vi "findChannelByAddress.vi"(8 "error in (no error)":errorcluster, 10 "channel_address":string, 11 "DeviceArray in":refnum<class "DeviceArray.lvclass">) -> (0 "error out":errorcluster, 1 "Channel.lvclass":refnum<class "Channel.lvclass">, 2 "device.lvclass":refnum<class "device.lvclass">, 3 "DeviceArray out":refnum<class "DeviceArray.lvclass">, 4 "found?":bool)   [LabVIEW 2011, in "Tools.lvlib" / "DatabaseHelpers.lvlib" / "DeviceArray.lvclass"]
uses:
  DeviceArray.lvclass
  Channel/Channel.lvclass
  device/device.lvclass
  DeviceArray.lvclass/DeviceArray.ctl
  ChannelArray/ChannelArray.lvclass
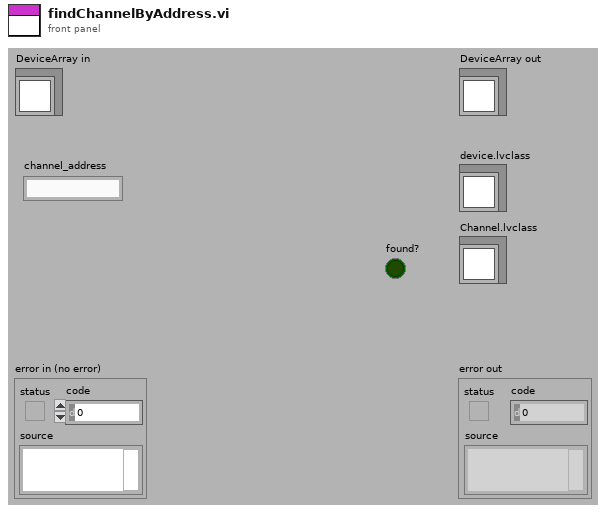
[diagram p1: front panel]
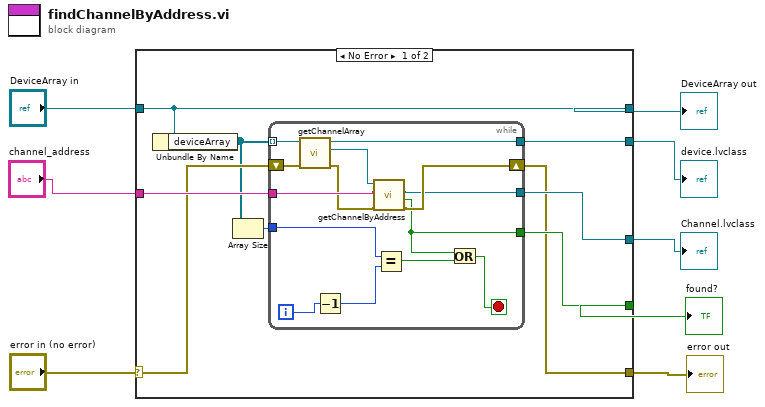
[diagram p0: block diagram]
diagram:
  n1 = case shown="No Error" "error in (no error)" {
    selector: "error in (no error)" -> [w15 w33]
    tunnel: [w9 w33] -> w3
    tunnel: [w17 w32] -> w7
    tunnel: "DeviceArray in" -> [w17 w32]
    tunnel: "channel_address" -> [w16 _]
    tunnel: [w12 _] -> w4
    tunnel: [w11 _] -> w6
    tunnel: [w10 _] -> w5
    frame No Error {
      n2 = Unbundle By Name(w17) -> ("deviceArray"=w14:refnum<class "device.lvclass">[])
      n3 = Array Size(array=w14) -> (size(s)=w13:i32)
      n4 = while {
        tunnel: w14 -> [w31] mode=indexing
        tunnel: w16 -> [w23]
        shift-right: [w20] -> w9
        shift-left: w15 -> [w30]
        tunnel: [w19] -> w10
        tunnel: [w29] -> w11
        tunnel: w13 -> [w27]
        tunnel: [w18] -> w12
        i -> [w28]
        stop <- w24 stop-if-true
        n5 = call "getChannelArray.vi"("error in (no error)"=w30, "device.lvclass in"=w31) -> ("error out"=w21:errorcluster, "ChannelArray.lvclass"=w22:refnum<class "ChannelArray.lvclass">, "device.lvclass out"=w29:refnum<class "device.lvclass">)  [unwired: 7 in]
        n6 = Decrement(x=w28) -> (x-1=w26:i32)
        n7 = call-dynamic "getChannelByAddress.vi"("error in (no error)"=w21, "channel_address"=w23, "ChannelArray in"=w22) -> ("error out"=w20:errorcluster, "found?"=w18:bool, "Channel"=w19:refnum<class "Channel.lvclass">)  [unwired: 5 in, 1 out]
        n8 = Equal?(x=w27, y=w26) -> (x = y?=w25:bool)
        n9 = Or(x=w18, y=w25) -> (x .or. y?=w24:bool)
      }
    }
    frame Error {
    }
  }
  "error out" <- w3
  "DeviceArray out" <- w7
  "Channel.lvclass" <- w5
  "device.lvclass" <- w6
  "found?" <- w4
